vi "cmc-worked-coordinate.vi"(8 "error in (no error)":errorcluster, 10 "Y Coordinate":dbl, 11 "X Coordinate":dbl) -> (0 "error out":errorcluster, 1 "Angle (degrees)":dbl, 2 "Angle (radians)":dbl, 3 "Radius":dbl)   [LabVIEW 2010]
doc: "This VI converts Cartesian x y coordinates to cylindrical polar coordinates. NOTE: both x and y units must match. The output radius is in the same units as x &y. The output angle is available as raidans and/or degrees fully resolved between all 4 quadrants.\n\ncreated by; Clair Cunningham\nRIT - Mechanical Engineering\nFall Quarter 2011"
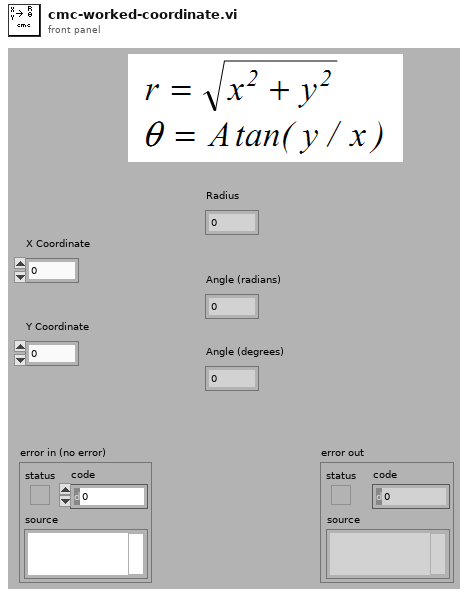
[diagram p1: front panel]
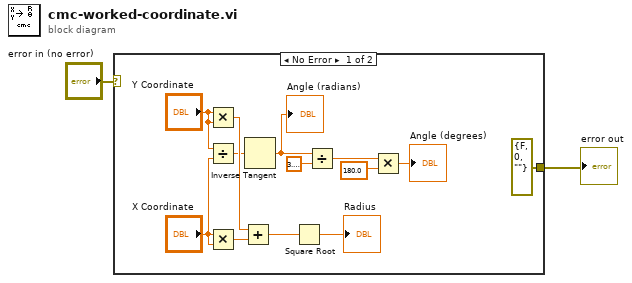
[diagram p0: block diagram]
diagram:
  n1 = case shown="No Error" "error in (no error)" {
    selector: "error in (no error)" -> [_ w16]
    tunnel: [errorcluster {"status"=FALSE, "code"=0, "source"=""} ("error out") w16] -> w1
    frame No Error {
      n2 = Multiply(x="Y Coordinate", y="Y Coordinate") -> (x*y=w12:dbl)
      n3 = Divide(x="Y Coordinate", y="X Coordinate") -> (x/y=w9:dbl)
      n4 = Multiply(x="X Coordinate", y="X Coordinate") -> (x*y=w13:dbl)
      n5 = Add(x=w12, y=w13) -> (x+y=w11:dbl)
      n6 = Inverse Tangent(1:w9) -> (0:w4:dbl)
      "Angle (radians)" <- w4
      n7 = Square Root(x=w11) -> (sqrt(x)=→"Radius":dbl)
      n8 = Divide(x=w4, y=3.141592653589793) -> (x/y=w8:dbl)
      n9 = Multiply(x=w8, y=180.0) -> (x*y=→"Angle (degrees)":dbl)
    }
    frame Error {
    }
  }
  "error out" <- w1
